vi "HRM-AQN-main.vi"(8 "error in (no error)":errorcluster, 11 "init cluster":T1) -> (0 "error out":errorcluster)   [LabVIEW 2020]
uses:
  init/HRM-init-cluster.ctl
  init/HRM-init-user_events.ctl
  process/HRM-process-Pulse settings.ctl
  init/HRM-init-Intial State.ctl
  init/HRM-init-hardware_selector.ctl
  HRM-AQN-input_clust.ctl
panel:
  out "pause AQN":bool
  in  "stop":bool
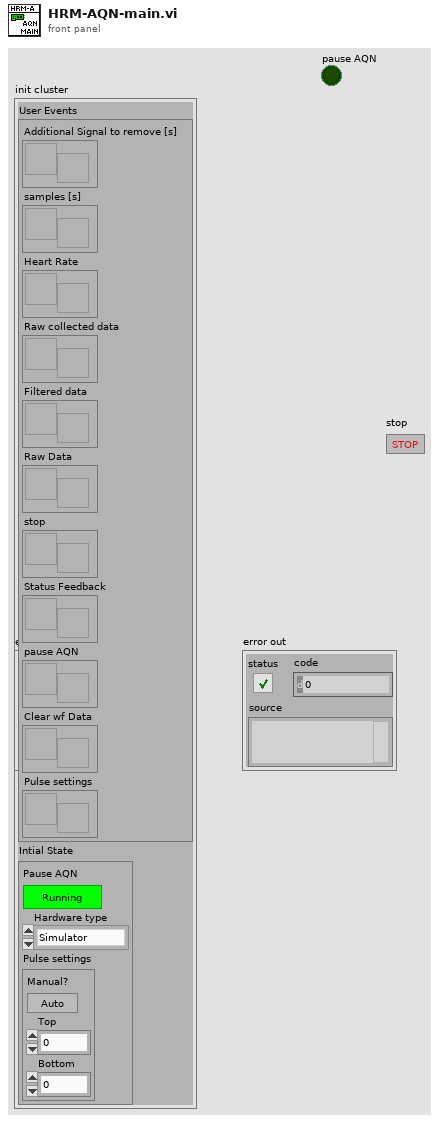
[diagram p1: front panel]
types:
  T1 = typedef "HRM-init-cluster.ctl" = cluster{"User Events":T2, "Intial State":T3}
  T2 = typedef "HRM-init-user_events.ctl" = cluster{"Additional Signal to remove [s]":refnum<user-event>, "samples [s]":refnum<user-event>, "Heart Rate":refnum<user-event>, "Raw collected data":refnum<user-event>, "Filtered data":refnum<user-event>, "Raw Data":refnum<user-event>, "stop":refnum<user-event>, "Status Feedback":refnum<user-event>, "pause AQN":refnum<user-event>, "Clear wf Data":refnum<user-event>, "Pulse settings":refnum<user-event>}
  T3 = typedef "HRM-init-Intial State.ctl" = cluster{"Pause AQN":bool, "Hardware type":T4, "Pulse settings":T5}
  T4 = typedef "HRM-init-hardware_selector.ctl" = enum16{"Simulator", "myDAQ", "Arduino", "Analog Discovery"}
  T5 = typedef "HRM-process-Pulse settings.ctl" = cluster{"Manual?":bool, "Top":dbl, "Bottom":dbl}
  T6 = typedef "HRM-AQN-input_clust.ctl" = cluster{"physical channels":tag, "myDAQ task":refnum<k21>}
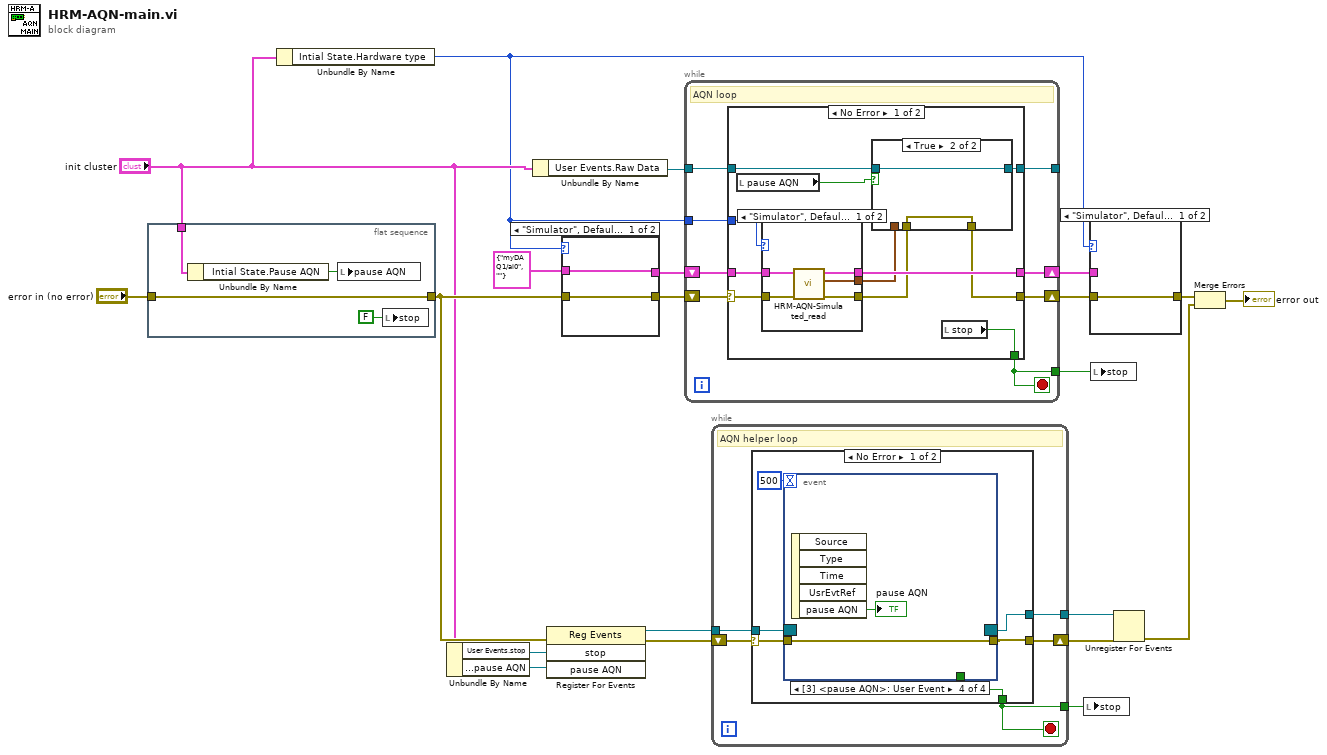
[diagram p0: block diagram]
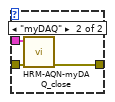
[diagram p2: hidden frame]
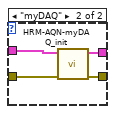
[diagram p3: hidden frame]
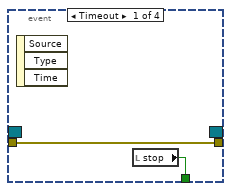
[diagram p4: hidden frame]
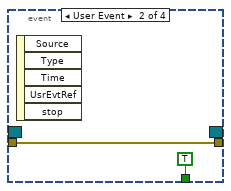
[diagram p5: hidden frame]
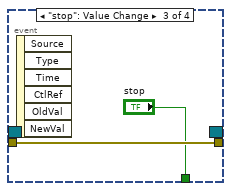
[diagram p6: hidden frame]
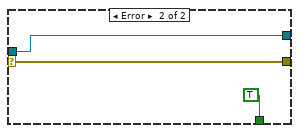
[diagram p7: hidden frame]
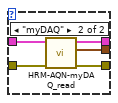
[diagram p8: hidden frame]
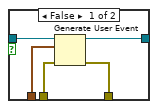
[diagram p9: hidden frame]
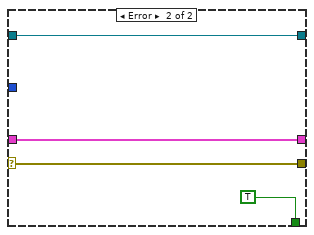
[diagram p10: hidden frame]
diagram:
  n1 = flat-sequence {
    tunnel: "error in (no error)" -> [w24]
    tunnel: [w24] -> w4
    tunnel: "init cluster" -> [w23]
    frame #0 {
      n2 = Unbundle By Name(w23) -> ("Intial State.Pause AQN"=w22:bool)
      n3 = local write "pause AQN"(w22) -> ()
      n4 = local write "stop"(FALSE ("stop")) -> ()
    }
  }
  n5 = Unbundle By Name("init cluster") -> ("Intial State.Hardware type"=w1:T4)
  n6 = Unbundle By Name("init cluster") -> ("User Events.stop"=w15:refnum<user-event>, "User Events.pause AQN"=w3:refnum<user-event>)
  n7 = Unbundle By Name("init cluster") -> ("User Events.Raw Data"=w19:refnum<user-event>)
  n8 = register-events(error in=w4, w15, w3) -> (reference out=w13:refnum<event-registration>, error out=w14:errorcluster)  [unwired: 1 in]
  n9 = case shown="\"Simulator\", Default" w1 {
    tunnel: [w26 w31] -> w20
    tunnel: [w27 w30] -> w17
    tunnel: T6 {"physical channels"="myDAQ1/ai0", "myDAQ task"=""} -> [w27 w29]
    tunnel: w4 -> [w26 w28]
    frame "Simulator", Default {
    }
    frame "myDAQ" {
      n10 = call "HRM-AQN-myDAQ_init.vi"("error in"=w28, "AQN cluster in"=w29) -> ("error out"=w31:errorcluster, "AQN cluster out"=w30:T6)  [unwired: 8 in]
    }
  }
  n11 = while {
    shift-right: [w38] -> w21
    shift-left: w20 -> [w39]
    shift-right: [w36] -> w18
    shift-left: w17 -> [w37]
    tunnel: w19 -> [w35]
    tunnel: [w34] -> _
    tunnel: [w33] -> w7
    tunnel: w1 -> [w32]
    stop <- w33 stop-if-true
    # "AQN loop"
    n12 = case shown="No Error" w39 {
      selector: w39 -> [w44 w71]
      tunnel: [w48 w71] -> w38
      tunnel: [w42 TRUE] -> w33
      tunnel: w37 -> [w50 w69]
      tunnel: [w49 w69] -> w36
      tunnel: w35 -> [w47 w68]
      tunnel: [w45 w68] -> w34
      tunnel: w32 -> [w40 _]
      frame No Error {
        n13 = local read "pause AQN"() -> (w41:bool)
        n14 = case shown="\"Simulator\", Default" w40 {
          tunnel: w50 -> [w55 w60]
          tunnel: [w52 w59] -> w49
          tunnel: [w53 w58] -> w46
          tunnel: w44 -> [w54 w57]
          tunnel: [w51 w56] -> w43
          frame "Simulator", Default {
            n15 = call "HRM-AQN-Simulated_read.vi"("error in (no error)"=w54, "AQN cluster in"=w55) -> ("error out"=w51:errorcluster, "data"=w53:waveform(dbl), "AQN cluster out"=w52:T6)  [unwired: 7 in]
          }
          frame "myDAQ" {
            n16 = call "HRM-AQN-myDAQ_read.vi"("error in (no error)"=w57, "AQN cluster in"=w60) -> ("error out"=w56:errorcluster, "data"=w58:waveform(dbl), "AQN cluster out"=w59:T6)  [unwired: 7 in]
          }
        }
        n17 = case shown="True" w41 {
          tunnel: [w65 w66] -> w48
          tunnel: w47 -> [w64 w67]
          tunnel: w46 -> [w63 _]
          tunnel: [w62 w67] -> w45
          tunnel: w43 -> [w61 w66]
          frame False {
            n18 = Generate User Event(user event=w64, event data cluster=w63, error in=w61) -> (user event out=w62:refnum<user-event>, error out=w65:errorcluster)  [unwired: 1 in]
          }
          frame True {
          }
        }
        n19 = local read "stop"() -> (w42:bool)
      }
      frame Error {
      }
    }
  }
  n20 = while {
    shift-right: [w75] -> w12
    shift-left: w14 -> [w76]
    tunnel: w13 -> [w74]
    tunnel: [w73] -> w11
    tunnel: [w72] -> w6
    stop <- w72 stop-if-true
    # "AQN helper loop"
    n21 = case shown="No Error" w76 {
      selector: w76 -> [w81 w93]
      tunnel: [w80 w93] -> w75
      tunnel: [w77 TRUE] -> w72
      tunnel: w74 -> [w82 w91]
      tunnel: [w79 w91] -> w73
      frame No Error {
        n22 = event shown="[3] <pause AQN>: User Event" {
          selector: w82 -> [_ _ _ _]
          dyn-events: [_ _ _ _] -> w79
          timeout: 500 -> [_ _ _ _]
          tunnel: w81 -> [w84 w86 w88 w90]
          tunnel: [w84 w86 w88 w90] -> w80
          tunnel: [w83 TRUE ("stop") "stop" _] -> w77
          event Timeout {
            n23 = event-data() -> ()  [unwired: 1 in, 3 out]
            n24 = local read "stop"() -> (w83:bool)
          }
          event User Event {
            n25 = event-data() -> ()  [unwired: 1 in, 5 out]
          }
          event "stop": Value Change {
            n26 = event-data() -> ()  [unwired: 1 in, 6 out]
          }
          event User Event {
            n27 = event-data() -> ("pause AQN"=→"pause AQN":bool)  [unwired: 1 in, 4 out]
          }
        }
      }
      frame Error {
      }
    }
  }
  n28 = local write "stop"(w6) -> ()
  n29 = case shown="\"Simulator\", Default" w1 {
    tunnel: w21 -> [w94 w97]
    tunnel: w18 -> [_ w96]
    tunnel: [w94 w95] -> w10
    frame "Simulator", Default {
    }
    frame "myDAQ" {
      n30 = call "HRM-AQN-myDAQ_close.vi"("error in (no error)"=w97, "AQN cluster in"=w96) -> ("error out"=w95:errorcluster)  [unwired: 9 in]
    }
  }
  n31 = local write "stop"(w7) -> ()
  n32 = Unregister For Events(event registration refnum=w11, error in=w12) -> (error out=w8:errorcluster)
  n33 = Merge Errors(w10, w8) -> (→"error out":errorcluster)
